vi "GetMovement.vi"(7 "Game Ticks":u32, 8 "error in (no error)":errorcluster, 10 "Move Speed":sgl, 11 "Input in":refnum<class "Input.lvclass">) -> (0 "error out":errorcluster, 2 "Move Vector":cluster{"[0]":sgl, "[1]":sgl, "[2]":sgl}, 3 "Input out":refnum<class "Input.lvclass">)   [LabVIEW 2015, in "Input.lvclass"]
uses:
  Input.lvclass
  Input.lvclass/Input.ctl
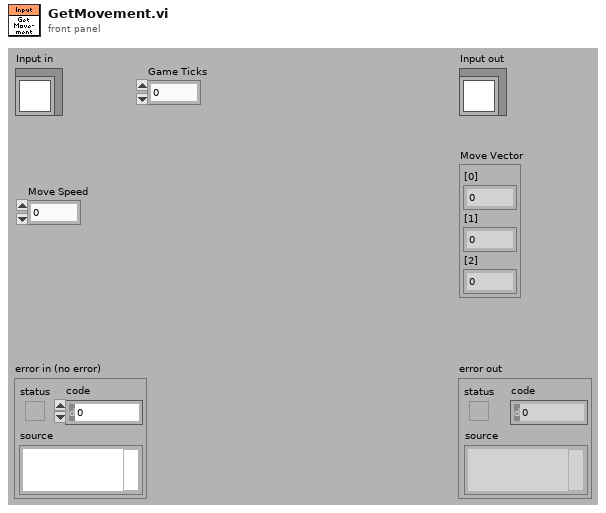
[diagram p1: front panel]
types:
  T1 = enum16{"0", "1", "2", "3", "4", "5", "6", "7", "8", "9", "A", "B", "C", "D", "E", "F", "G", "H", "I", "J", "K", "L", "M", "N", "O", "P", "Q", "R", "S", "T", "U", "V", "W", "X", "Y", "Z", "F1", "F2", "F3", "F4", "F5", "F6", "F7", "F8", "F9", "F10", "F11", "F12", "F13", "F14", "F15", "ADD", "BACK", "BACKSLASH", "CAPITAL", "COMMA", "DECIMAL", "DELETE", "DIVIDE", "DOWN", "END", "EQUALS", "ESCAPE", "GRAVE (`)", "HOME", "INSERT", "LBRACKET", "LCONTROL", "LEFT", "L ALT", "LSHIFT", "LWIN", "MINUS", "MULTIPLY", "NEXT", "NUMLOCK", "NUMPAD_0", "NUMPAD_1", "NUMPAD_2", "NUMPAD_3", "NUMPAD_4", "NUMPAD_5", "NUMPAD_6", "NUMPAD_7", "NUMPAD_8", "NUMPAD_9", "PAUSE", "PERIOD", "PRIOR (PG UP)", "RBRACKET", "RCONTROL", "RETURN", "RIGHT", "R ALT", "RSHIFT", "RWIN", "SCROLL", "SEMICOLON", "SLASH", "SPACE", "SUBTRACT", "TAB", "UP", "ENTER (num pad)", "' (quote)"}[]
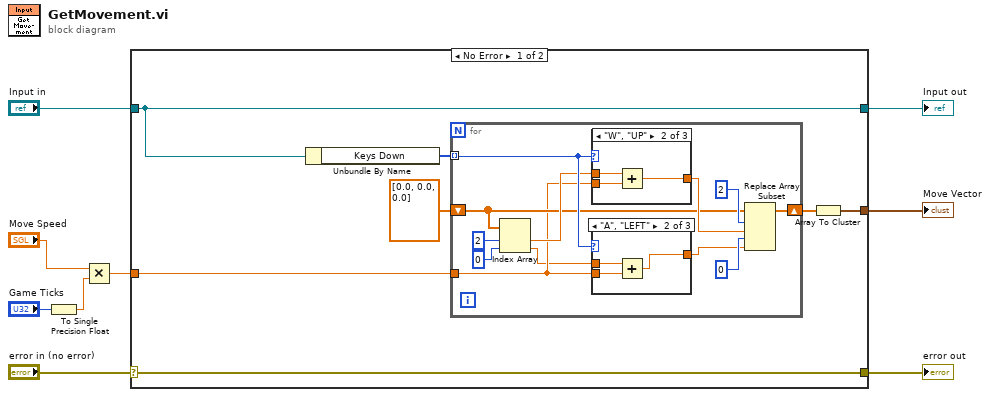
[diagram p0: block diagram]
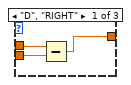
[diagram p2: hidden frame]
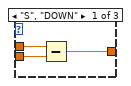
[diagram p4: hidden frame]
diagram:
  n1 = To Single Precision Float(number="Game Ticks") -> (single precision float=w2:sgl)
  n2 = Multiply(x="Move Speed", y=w2) -> (x*y=w5:sgl)
  n3 = case shown="No Error" "error in (no error)" {
    selector: "error in (no error)" -> [w16 w44]
    tunnel: [w16 w44] -> w8
    tunnel: [w15 w43] -> w6
    tunnel: "Input in" -> [w15 w43]
    tunnel: w5 -> [w10 _]
    tunnel: [w13 _] -> w4
    frame No Error {
      n4 = Unbundle By Name(w15) -> ("Keys Down"=w12:T1)
      n5 = for {
        tunnel: w12 -> [w28] mode=indexing
        tunnel: w10 -> [w20]
        shift-right: [w23] -> w11
        shift-left: sgl[] [0.0, 0.0, 0.0] -> [w21]
        n6 = Index Array(array=w21, index #1=2 ("index"), index #2=0 ("index")) -> (element #1=w22:sgl, element #2=w17:sgl)
        n7 = case shown="\"W\", \"UP\"" w28 {
          tunnel: [w36 w41 w42] -> w24
          tunnel: w22 -> [w37 w40 w42]
          tunnel: w20 -> [w38 w39 _]
          frame "S", "DOWN" {
            n8 = Subtract(x=w37, y=w38) -> (x-y=w36:sgl)
          }
          frame "W", "UP" {
            n9 = Add(x=w40, y=w39) -> (x+y=w41:sgl)
          }
          frame Default {
          }
        }
        n10 = case shown="\"A\", \"LEFT\"" w28 {
          tunnel: w17 -> [w30 w34 w35]
          tunnel: w20 -> [w31 w33 _]
          tunnel: [w29 w32 w35] -> w25
          frame "D", "RIGHT" {
            n11 = Subtract(x=w30, y=w31) -> (x-y=w29:sgl)
          }
          frame "A", "LEFT" {
            n12 = Add(x=w34, y=w33) -> (x+y=w32:sgl)
          }
          frame Default {
          }
        }
        n13 = Replace Array Subset(array=w21, new element #1=w24, index #1=2 ("index"), new element #2=w25, index #2=0 ("index")) -> (w23:sgl[])
      }
      n14 = Array To Cluster(array=w11) -> (cluster=w13:cluster{"[0]":sgl, "[1]":sgl, "[2]":sgl})
    }
    frame Error {
    }
  }
  "error out" <- w8
  "Input out" <- w6
  "Move Vector" <- w4
